vi "agilent_resistances_to_temps.vi"(1 "Therm Coefs":string[][](array[string])=[["Locn", "Probe", "Channel", "Res to Temp Equation", "CalDate"], ["Cell", "M5", "101", "197.4556-51.4464*log(x)", "canned"], ["Acid", "V1", "102", "197.4556-51.4464*log(x)", "canned"], ["Brt", "S4", "103", "197.4556-51.4464*log(x)", "canned"], ["Room", "A3", "104", "197.4556-51.4464*log(x)", "canned"]], 2 "Resistance":dbl) -> (0 "Cell T":dbl)   [LabVIEW 2010]
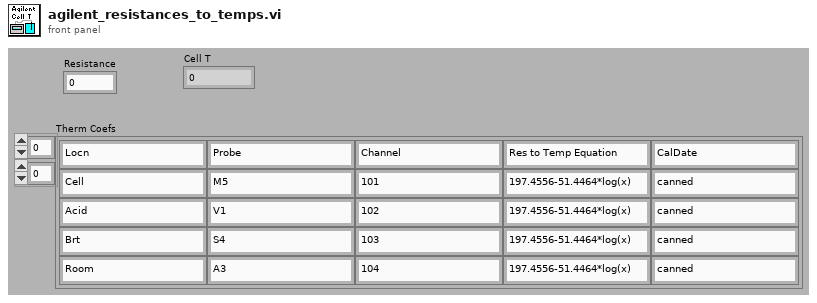
[diagram p1: front panel]
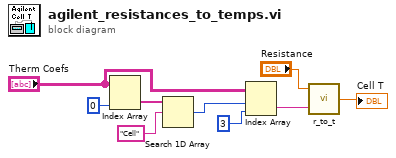
[diagram p0: block diagram]
diagram:
  n1 = Index Array(array="Therm Coefs", index (col)=0 ("disabled index (col)")) -> (element=w8:string[])  [unwired: 1 in]
  n2 = Search 1D Array(1D array=w8, element="Cell") -> (index of element=w4:i32)  [unwired: 1 in]
  n3 = Index Array(array="Therm Coefs", index (row)=w4, index (col)=3 ("disabled index (col)")) -> (element=w5:string)
  n4 = call "r_to_t.vi"("T equation"=w5, "Resistance"="Resistance") -> ("Temperature"=→"Cell T":dbl)  [unwired: 1 in]
